vi "Execute.vi"(8 "error in (no error)":errorcluster, 11 "Node in":refnum<class "bt_Send_Notifier.lvclass">) -> (0 "error out":errorcluster, 1 "Status":T1, 3 "Node out":refnum<class "bt_Send_Notifier.lvclass">)   [LabVIEW 2021, in "BT.lvlib" / "bt_Send_Notifier.lvclass"]
uses:
  bt_Send_Notifier.lvclass
  C:/Users/Tim/Documents/GitHub/LV_Behaviour_Tree/Source/Support/Nodes/Leaves/Synch/With Values/Send/bt_Send_Synch_WithValues.lvclass
  abs_Node/Status.ctl
  With Values/Send/bt_Send_Synch_WithValues.lvclass/bt_Send_Synch_WithValues.ctl
  bt_Send_Notifier.lvclass/bt_Send_Notifier.ctl
  With Values/Send/Properties/Read Values.vi
  abs_Node/bt_Node.lvclass
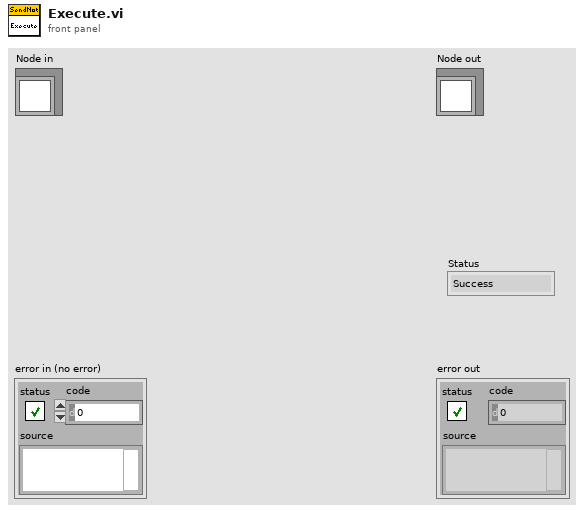
[diagram p1: front panel]
types:
  T1 = typedef "BT.lvlib/bt_Node.lvclass/Status.ctl" = enum16{"Success", "Failure", "Running"}
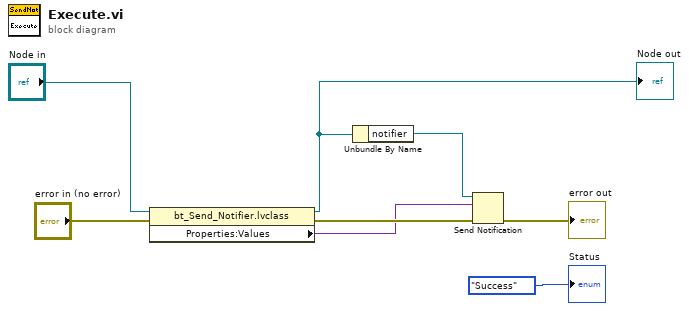
[diagram p0: block diagram]
diagram:
  n1 = property class="bt_Send_Notifier.lvclass"(reference="Node in", error in="error in (no error)") -> (reference out=w5:refnum<class "bt_Send_Notifier.lvclass">, error out=w4:errorcluster, "Properties:Values"=w1:variant)
  "Node out" <- w5
  n2 = Unbundle By Name(w5) -> ("notifier"=w8:refnum<notifier>)
  n3 = Send Notification(notification=w1, notifier=w8, error in (no error)=w4) -> (error out=→"error out":errorcluster)  [unwired: 1 out]
  "Status" <- Status."Success" ("Status")
